vi "Save Snippets.vi"() -> ()   [LabVIEW 2016]
uses:
  CNN/Training/TrainerBase/TrainerBase.lvclass
  CNN/Volume/Volume.lvclass
  C:/Users/DUE/Desktop/Projects/CAIRO/Open Source Projects/CNN/dev/CNN/IVolume/IVolume.lvclass
panel:
  in  "Number of Sample":i32
  in  "Data Sample":dbl[][](array[numeric])
  in  "Sample Target":i32[](array[numeric])
  in  "CNN.lvlib:TrainerBase.lvclass":refnum<class "TrainerBase.lvclass">
  out "error out":errorcluster
  out "avLoss":dbl
  in  "error in (no error)":errorcluster
  out "CNN.lvlib:TrainerBase.lvclass 2":refnum<class "TrainerBase.lvclass">
  out "Image Path":path
  in  "vi path":path
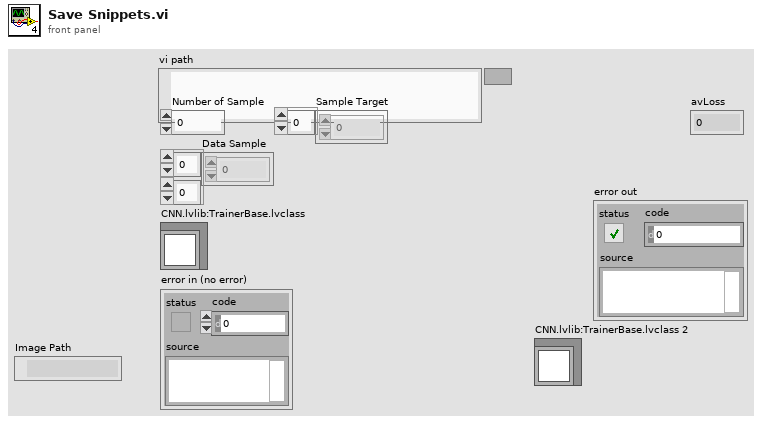
[diagram p1: front panel]
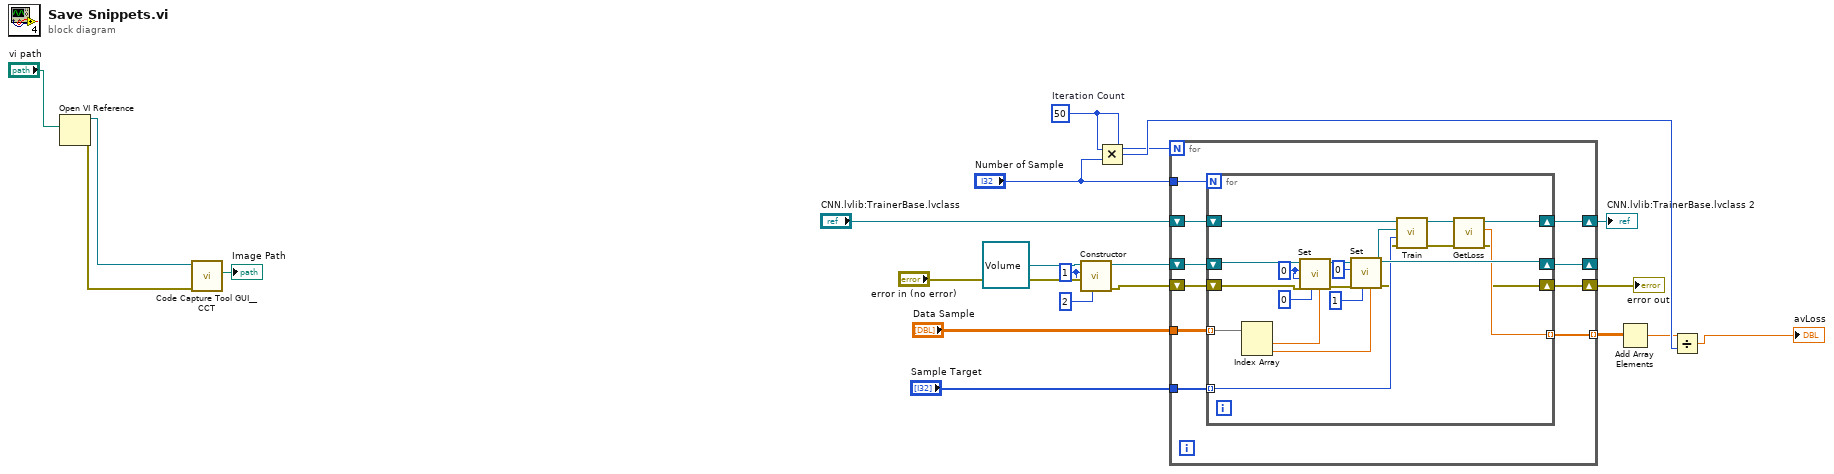
[diagram p0: block diagram]
diagram:
  w13 = 50  # Iteration Count
  w2 = 1 ("width")
  n1 = Open VI Reference(vi path="vi path") -> (vi reference=w19:refnum<vi>, error out=w18:errorcluster)  [unwired: 5 in]
  n2 = call <vilib>:"Code Capture Tool GUI__CCT.vi"("error in (no error)"=w18, "VI to Capture"=w19) -> ("Image Path"=→"Image Path":path)  [unwired: 7 in, 2 out]
  n3 = call-dynamic "Constructor.vi"("depth"=2, "error in (no error)"="error in (no error)", "height"=w2, "width"=w2, "Volume in"=refnum<class "Volume.lvclass"> refnum ("CNN.lvlib:Volume.lvclass")) -> ("error out"=w7:errorcluster, "Volume out"=w4:refnum<class "Volume.lvclass">)  [unwired: 5 in]
  n4 = Multiply(x=w13, y="Number of Sample") -> (x*y=w14:i32)
  n5 = for {
    N: w13 -> [_]
    shift-right: [w30] -> _
    shift-left: w4 -> [w31]
    shift-right: [w28] -> w17
    shift-left: "CNN.lvlib:TrainerBase.lvclass" -> [w29]
    tunnel: "Number of Sample" -> [w27]
    tunnel: "Data Sample" -> [w26]
    shift-right: [w24] -> w8
    shift-left: w7 -> [w25]
    tunnel: [w23] -> w9 mode=indexing
    tunnel: "Sample Target" -> [w22]
    n6 = for {
      N: w27 -> [_]
      shift-right: [w46] -> w30
      shift-left: w31 -> [w50]
      shift-right: [w37] -> w28
      shift-left: w29 -> [w51]
      tunnel: w26 -> [w49] mode=indexing
      shift-right: [w32] -> w24
      shift-left: w25 -> [w39]
      tunnel: [w36] -> w23 mode=indexing
      tunnel: w22 -> [w35] mode=indexing
      w45 = 0 ("x")
      n7 = Index Array(array=w49) -> (element #1=w44:dbl, element #2=w43:dbl)  [unwired: 2 in]
      n8 = call-dynamic "Set.vi"("v"=w44, "d"=0, "error in (no error)"=w39, "y"=w45, "x"=w45, "Volume in"=w50) -> ("error out"=w48:errorcluster, "Volume out"=w47:refnum<class "Volume.lvclass">)  [unwired: 4 in]
      n9 = call-dynamic "Set.vi"("v"=w43, "d"=1, "error in (no error)"=w48, "x"=0, "Volume in"=w47) -> ("error out"=w33:errorcluster, "Volume out"=w46:refnum<class "Volume.lvclass">)  [unwired: 5 in]
      n10 = call-dynamic "Train.vi"("error in (no error)"=w33, "y"=w35, "CNN.lvlib:IVolume.lvclass"=w46, "TrainerBase in"=w51) -> ("error out"=w34:errorcluster, "TrainerBase out"=w38:refnum<class "TrainerBase.lvclass">)  [unwired: 6 in]
      n11 = call-dynamic "GetLoss.vi"("error in (no error)"=w34, "TrainerBase in"=w38) -> ("error out"=w32:errorcluster, "Loss"=w36:dbl, "TrainerBase out"=w37:refnum<class "TrainerBase.lvclass">)  [unwired: 7 in]
    }
  }
  "error out" <- w8
  "CNN.lvlib:TrainerBase.lvclass 2" <- w17
  n12 = Add Array Elements(numeric array=w9) -> (sum=w11:dbl)
  n13 = Divide(x=w11, y=w14) -> (x/y=→"avLoss":dbl)
